vi "Test Pass if Expected API Call Made Using Tolerant Comparator.vi"(8 "error in (no error)":errorcluster, 11 "Test Case In":refnum<class "Pure Mock One or More Expectation Test.lvclass">) -> (0 "error out":errorcluster, 3 "Test Case Out":refnum<class "Pure Mock One or More Expectation Test.lvclass">)   [LabVIEW 2020, in "Pure Mock One or More Expectation Test.lvclass"]
uses:
  Pure Mock One or More Expectation Test.lvclass
  C:/Program Files (x86)/National Instruments/LabVIEW 2020/vi.lib/Astemes/LUnit/Test Case.lvclass
  source/Comparators/Tolerant Numeric Argument Comparator/Tolerant Numeric Argument Comparator.lvclass
  C:/git/astemes-lmock/source/Core/Comparator/Comparator.lvclass
  Test Doubles/Test Interface Responsive Mock/Test Interface Responsive Mock.lvclass
  C:/git/astemes-lmock/source/Core/Mock/Mock.lvclass
  Pure Mock One or More Expectation Test.lvclass/Pure Mock One or More Expectation Test.ctl
  Expectation Test/Responsive Mock Expectation Test.lvclass
  source/Expectations/One or More/One or More.lvclass
  Test Doubles/Test Interface Pure Mock/Test Interface Pure Mock.lvclass
  C:/git/astemes-lmock/source/Framework/Pure Mock/Pure Mock.lvclass
  C:/git/astemes-lmock/tests/Test Doubles/Test Interface Pure Mock/Test Interface Pure Mock.lvclass
  C:/git/astemes-lmock/tests/Test Doubles/Test Interface/Test Interface.lvclass
  C:/git/astemes-lmock/source/Comparators/Tolerant Numeric Argument Comparator/Tolerant Numeric Argument Comparator.lvclass
  C:/git/astemes-lmock/tests/Expectation Test/Expectation Test.lvclass
  C:/Program Files (x86)/National Instruments/LabVIEW 2020/vi.lib/Astemes/LUnit/LUnit Runnable.lvclass
  C:/git/astemes-lmock/tests/Pure Mock One or More Expectation Test/Pure Mock One or More Expectation Test.lvclass
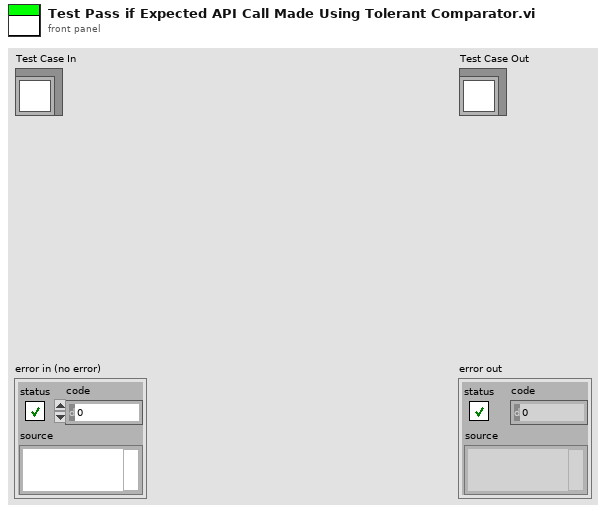
[diagram p1: front panel]
types:
  T1 = enum16{"", "Passed", "Failed", "Error", "Skipped", "Setup Error", "Broken", "Teardown Error"}
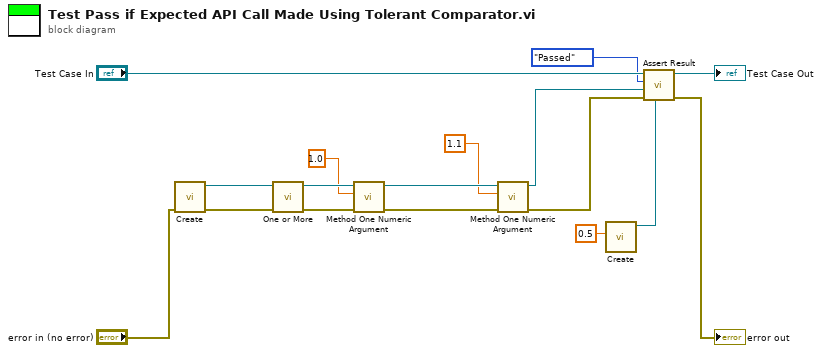
[diagram p0: block diagram]
diagram:
  n1 = call "Create.vi"("error in (no error)"="error in (no error)") -> ("error out"=w16:errorcluster, "Test Interface Mock Out"=w17:refnum<class "Test Interface Pure Mock.lvclass">)  [unwired: 9 in]
  n2 = call "One or More.vi"("error in (no error)"=w16, "Mock in"=w17) -> ("error out"=w14:errorcluster, "Mock out"=w15:refnum<class "Test Interface Pure Mock.lvclass">)  [unwired: 8 in]
  n3 = call-dynamic "Method One Numeric Argument.vi"("error in (no error)"=w14, "Numeric"=1.0, "Test Interface Mock In"=w15) -> ("error out"=w13:errorcluster, "Test Interface Mock Out"=w6:refnum<class "Test Interface Pure Mock.lvclass">)  [unwired: 7 in]
  n4 = call-dynamic "Method One Numeric Argument.vi"("error in (no error)"=w13, "Numeric"=1.1, "Test Interface Mock In"=w6) -> ("error out"=w7:errorcluster, "Test Interface Mock Out"=w5:refnum<class "Test Interface Pure Mock.lvclass">)  [unwired: 7 in]
  n5 = call "Create.vi"("Tolerance"=0.5) -> ("Tolerant Numeric Comparator Out"=w1:refnum<class "Tolerant Numeric Argument Comparator.lvclass">)  [unwired: 9 in, 1 out]
  n6 = call "Assert Result.vi"("Comparator"=w1, "error in (no error)"=w7, "Mock"=w5, "Status"=T1."Passed", "LUnit Test Case In"="Test Case In") -> ("error out"=→"error out":errorcluster, "LUnit Test Case Out"=→"Test Case Out":refnum<class "Pure Mock One or More Expectation Test.lvclass">)  [unwired: 5 in]
